vi "Set SLSC Switch Resource.vi"(8 "error in (no error)":errorcluster, 10 "Resource":string, 11 "SLSC Switch Custom Device Ref in":T1 format="%.0x") -> (0 "error out":errorcluster, 3 "SLSC Switch Custom Device Ref out":T1 format="%.0x")   [LabVIEW 2017, in "SLSC Switch Scripting.lvlib"]
uses:
  SLSC Switch Scripting.lvlib
  <vilib>/NI Veristand/Custom Device API/Custom Device Item Ref.ctl
  Shared/Routing and Faulting Hardware API/Routing and Faulting Hardware API.lvlib
  <vilib>/NI Veristand/Custom Device API/Custom Device API.lvlib
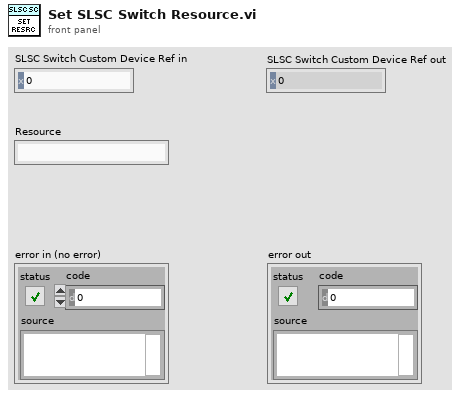
[diagram p1: front panel]
types:
  T1 = typedef "Custom Device API.lvlib/Custom Device Item Ref.ctl" = u64
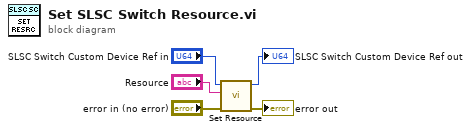
[diagram p0: block diagram]
diagram:
  n1 = call "Set Resource.vi"("error in (no error)"="error in (no error)", "Resource"="Resource", "Hardware Ref in"="SLSC Switch Custom Device Ref in") -> ("error out"=→"error out":errorcluster, "Hardware Ref out"=→"SLSC Switch Custom Device Ref out":T1)  [unwired: 7 in]
